vi "getRfState.vi"(8 "error in (no error)":errorcluster, 9 "state_name":string, 10 "channel_name":string, 11 "ChannelArray in":refnum<class "ChannelArray.lvclass">) -> (0 "error out":errorcluster, 2 "rf_state":T1, 3 "ChannelArray out":refnum<class "ChannelArray.lvclass">)   [LabVIEW 2011, in "Tools.lvlib" / "DatabaseHelpers.lvlib" / "ChannelArray.lvclass"]
uses:
  ChannelArray.lvclass
  Channel/RfOutputChannel/RfOutputChannel.lvclass
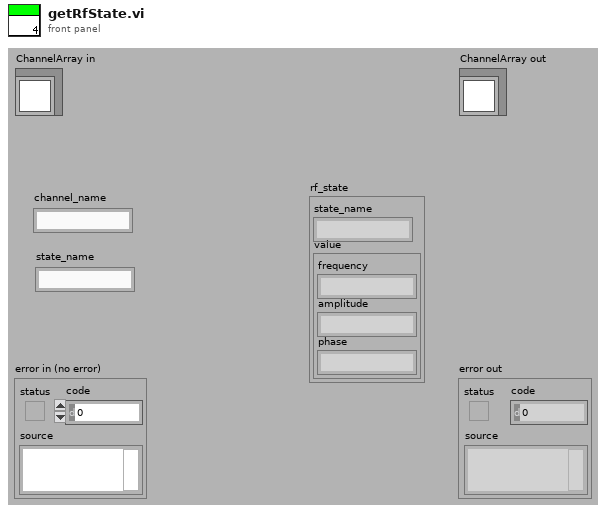
[diagram p1: front panel]
types:
  T1 = cluster{"state_name":string, "value":cluster{"frequency":string, "amplitude":string, "phase":string}}
  T2 = cluster{"state_name":string, "value":cluster{"frequency":string, "amplitude":string, "phase":string}}[]
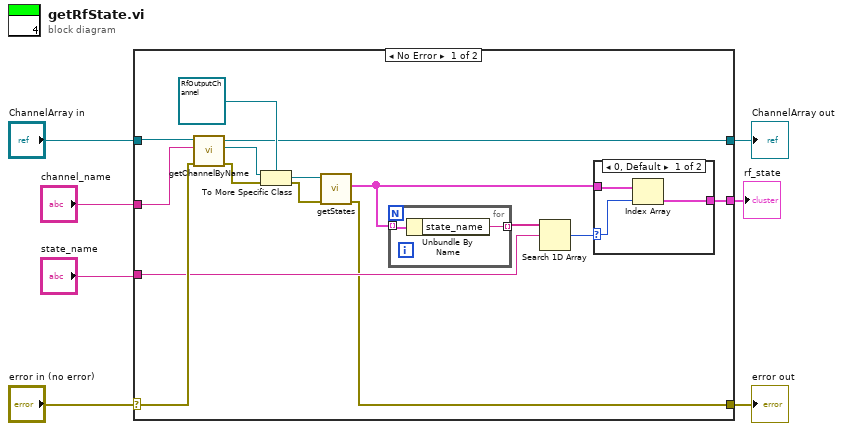
[diagram p0: block diagram]
diagram:
  n1 = case shown="No Error" "error in (no error)" {
    selector: "error in (no error)" -> [w20 w29]
    tunnel: [w8 w29] -> w6
    tunnel: [w9 w28] -> w4
    tunnel: "ChannelArray in" -> [w22 w28]
    tunnel: "channel_name" -> [w21 _]
    tunnel: "state_name" -> [w13 _]
    tunnel: [w10 _] -> w1
    frame No Error {
      n2 = call-dynamic "getChannelByName.vi"("error in (no error)"=w20, "channel_name"=w21, "ChannelArray in"=w22) -> ("error out"=w15:errorcluster, "Channel"=w16:refnum<class "Channel.lvclass">, "ChannelArray out"=w9:refnum<class "ChannelArray.lvclass">)  [unwired: 5 in, 1 out]
      n3 = To More Specific Class(target class=refnum<class "RfOutputChannel.lvclass"> refnum ("RfOutputChannel in"), reference=w16, error in=w15) -> (specific class reference=w18:refnum<class "RfOutputChannel.lvclass">, error out=w19:errorcluster)
      n4 = call "getStates.vi"("error in (no error)"=w19, "RfOutputChannel in"=w18) -> ("error out"=w8:errorcluster, "states"=w11:T2)  [unwired: 7 in, 1 out]
      n5 = for {
        tunnel: w11 -> [w27] mode=indexing
        tunnel: [w26] -> w14 mode=indexing
        n6 = Unbundle By Name(w27) -> ("state_name"=w26:string)
      }
      n7 = Search 1D Array(1D array=w14, element=w13) -> (index of element=w12:i32)  [unwired: 1 in]
      n8 = case shown="0, Default" w12 {
        selector: w12 -> [w25 _]
        tunnel: w11 -> [w24 _]
        tunnel: [w23 _] -> w10
        frame 0, Default {
          n9 = Index Array(array=w24, index=w25) -> (element=w23:T1)
        }
        frame -1 {
        }
      }
    }
    frame Error {
    }
  }
  "error out" <- w6
  "ChannelArray out" <- w4
  "rf_state" <- w1
